vi "3D Acquisition.vi"(6 "remote cmd":T1) -> (7 "remote response":T1)   [LabVIEW 2023, in "CX Labview Wrapper.lvlib"]
uses:
  CX Labview Wrapper.lvlib
  <vilib>/userDefined/High Color/IMAQdx.ctl
  Controls/2D Camsettings.ctl
  Controls/3D Camsettings.ctl
  <extravilib>/ChannelInstances/Messenger-t'Message Queue.lvlib-Message Cluster.ctl'/))Channel.ctl
  modules/cmh-library/Message Queue/Message Cluster.ctl
  Modules/imaqdx-classes/imaqdx/C5/C5.lvclass
  D:/gitlab/thermography-acquisition/thermography-acquisition/modules/imaqdx-classes/imaqdx/Camera/GigE Camera.lvclass
  9e623b8b-350b-4dac-bc7c-d4b869b38778.vi
  5610718c-0c97-4d59-862b-e515b301dfbc.vi
  16968268-87fa-4872-9799-b0272440c818.vi
  4f413283-1e67-4ee1-b33a-2c7c3799b1f0.vi
  <extravilib>/ChannelInstances/Messenger-t'Message Queue.lvlib-Message Cluster.ctl'/Write With Abort.vi
  <extravilib>/ChannelInstances/Event Messenger-bool/Instantiate.vi
  <extravilib>/ChannelInstances/Event Messenger-bool/))Channel.vi
  <extravilib>/ChannelInstances/Messenger-t'Message Queue.lvlib-Message Cluster.ctl'/Endpoint.vi
  modules/cmh-library/Message Queue/Enqueue Multiple Messages.vi
  gitlab/thermography-acquisition/thermography-acquisition/modules/imaqdx-classes/imaqdx/Camera/Write Attributes from VArrays Cluster.vi
  Modules/cmh-library/Message Queue.lvlib
  gitlab/thermography-acquisition/thermography-acquisition/modules/imaqdx-classes/imaqdx/Camera/GigE Camera.lvclass
  modules/cmh-library/Message Queue Helper.lvlib
  <extravilib>/ChannelInstances/Event Messenger-bool.lvlib
  <vilib>/addons/_JKI.lib/Serialization/JSON/JKI JSON Serialization.lvlib
  D:/git/CX-LabVIEW-Wrapper/VI/Modules/imaqdx-classes/imaqdx/3D/3D.lvclass
  D:/git/CX-LabVIEW-Wrapper/VI/Modules/imaqdx-classes/imaqdx/C5/C5.lvclass
  <extravilib>/ChannelInstances/Messenger-t'Message Queue.lvlib-Message Cluster.ctl'.lvlib
panel:
  in  "Close Button":bool
  out "success":i32
  out "Initialized":bool
  in  "3D Cam":T2="C5"
  out "Log":string
  out "error out":errorcluster
  in  "Main Tab Control":enum32{"3D Image", "2D Image", "All Settings"}(tab)
  in  "Open 3D Image":bool caption="Open Image"
  in  "Save Pointcloud":bool
  in  "Save 3D Settings":bool caption="Save"
  in  "Apply 3D Settings":bool caption="Apply"
  in  "Channel":u16(ring) items=["DC0", "DC1", "DC2"]
  out "FrameRate":dbl caption="FrameRate [Hz]" format="%#.2g"
  out "Traversal [mm]":dbl format="%#.2g"
  in  "Acquire 3D Button":bool caption="Acquire 3D"
  in  "Save 3D Image":bool caption="Save Image"
  in  "3D Mode Camsettings":T3={"CameraMode"=0, "ProfilesPerFrame"=0, "ExposureTimeAbs"=9000, "FramePeriod"=0, "ProfileTriggerMode"=0, "OutputImageType"=0, "FIR"=FALSE, "AcquisitionMode"=0, "AcquisitionFrameCount"=0, "AOIThreshold"=0, "AOIHeight"=0, "NumSubPixel"=0, "TriggerDivider"=0, "EnableDC0"=FALSE, "EnableDC1"=FALSE, "EnableDC2"=FALSE, "Timeout"=0} {"OutputImageType" items=["Auto"=2147483647, "Grayscale (U8)"=0, "Grayscale (I16)"=1, "Grayscale (U16)"=7, "RGB (U32)"=4, "RGB (U64)"=6]; "ProfileTriggerMode" items=["Free-Run", "Camera Input1", "Camera Input2", "Encoder/Resolver Interface RS422"]; "CameraMode" items=["Image Mode (IMG)"=0, "3D FIR Peak (PEAK)"=4, "3D Center of Gravity (COG)"=3, "3D Threshold (TRSH)"=1, "3D Maximum Intensity (MAX)"=2]; "AcquisitionMode" items=["Continuous", "Single Frame", "Multiple Frame"]}
  out "Depth Image":u16[][](graph)
  in  "CalibId":string="cal0"
  in  "Save 2D Settings":bool
  out "Processed FPS":dbl
  out "Acquired FPS":dbl
  in  "2D Play Button":bool
  in  "2D Stop Button":bool
  in  "Save Image":bool
  in  "2D Mode Camsettings":T4={"CameraMode"=0, "ExposureTimeAbs"=0, "AOIThreshold"=0.0, "FramePeriod"=0, "ProfileTriggerMode"=0, "OutputImageType"=7, "AcquisitionMode"=0, "Timeout"=1000, "EnableDC0"=TRUE} {"AcquisitionMode" items=["Continuous", "Single Frame", "Multiple Frame"]; "OutputImageType" items=["Auto"=2147483647, "Grayscale (U8)"=0, "Grayscale (I16)"=1, "Grayscale (U16)"=7, "RGB (U32)"=4, "RGB (U64)"=6]; "ProfileTriggerMode" items=["Free-Run", "Camera Input1", "Camera Input2", "Encoder/Resolver Interface RS422"]; "CameraMode" items=["Image Mode (IMG)"=0, "3D FIR Peak (PEAK)"=4, "3D Center of Gravity (COG)"=3, "3D Threshold (TRSH)"=1, "3D Maximum Intensity (MAX)"=2]}
  out "Intensity Image":u16[][](graph)
  out "2D Detail Graph":u16[][](graph)
  in  "Tab Control Pams":T5(tab)
  in  "U32 Value Control":u32(slide) step=1 scale=0.0..4294967295.0 scale format="%.0e"
  in  "DBL Value Control":dbl(slide) min=0.0 max=1023.0 step=1.0 scale=0.0..1023.0
  in  "String Value Control":string
  in  "Enum Value Control":u32(ring) items=["Image Mode (IMG)", "3D FIR Peak (PEAK)", "3D Center of Gravity (COG)", "3D Threshold (TRSH)", "3D Maximum Intensity (MAX)"]
  in  "Boolean Value Control":bool
  in  "Command Value Control":bool
  in  "Attribute Tree":string(tree)
  out "Tooltip":string
  out "Units":string
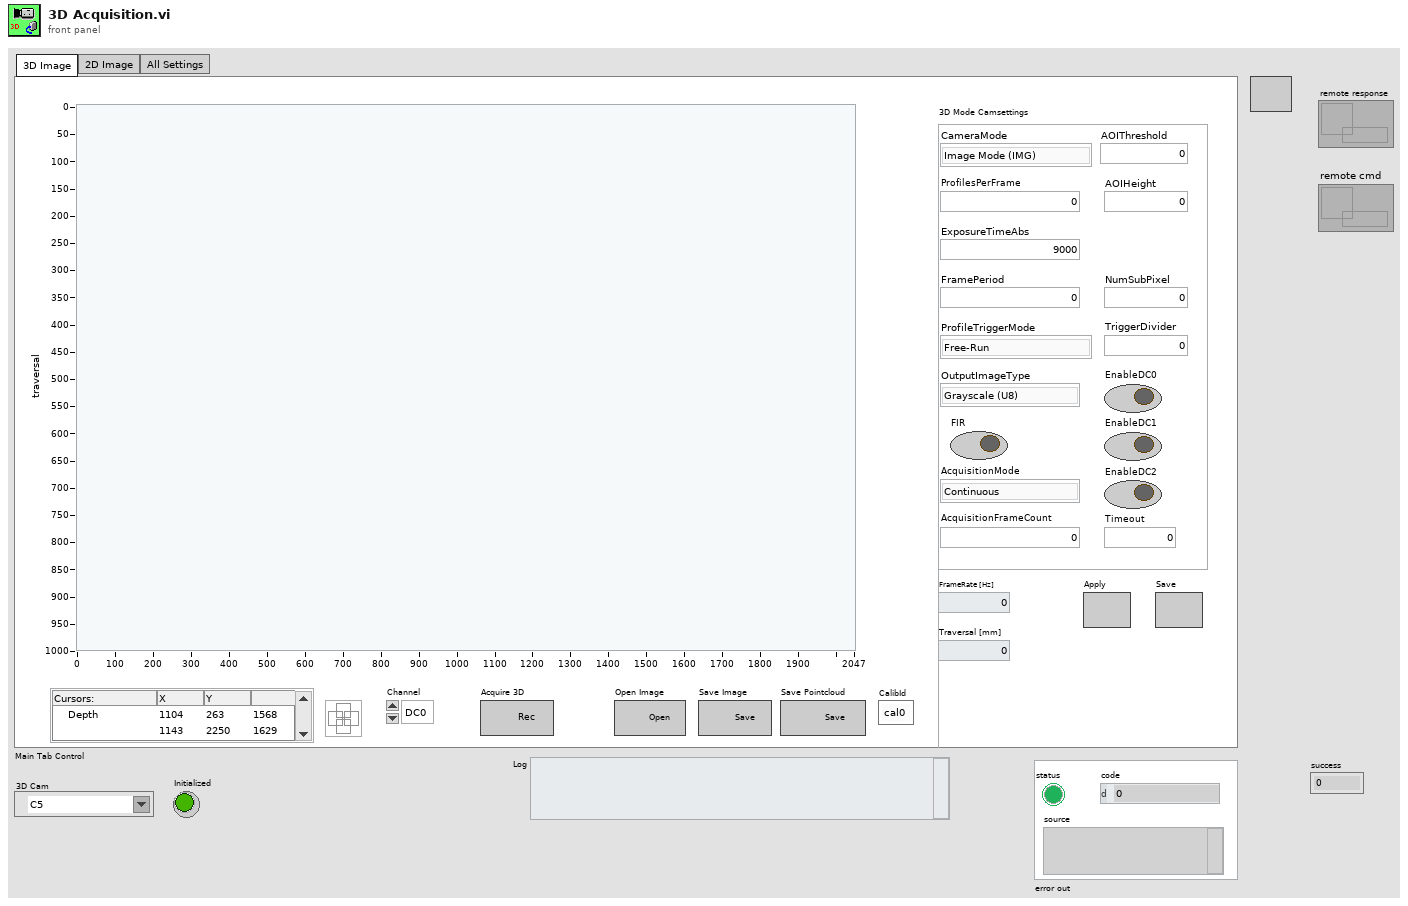
[diagram p1: front panel]
types:
  T1 = typedef "Messenger-t'Message Queue.lvlib-Message Cluster.ctl'.lvlib/))Channel.ctl" = refnum<queue>
  T2 = typedef "IMAQdx.ctl" = refnum<k21>
  T3 = typedef "CX Labview Wrapper.lvlib/3D Camsettings.ctl" = cluster{"CameraMode":u32, "ProfilesPerFrame":i64, "ExposureTimeAbs":i64, "FramePeriod":i64, "ProfileTriggerMode":u32, "OutputImageType":u32, "FIR":bool, "AcquisitionMode":u32, "AcquisitionFrameCount":i64, "AOIThreshold":i64, "AOIHeight":i64, "NumSubPixel":i64, "TriggerDivider":i64, "EnableDC0":bool, "EnableDC1":bool, "EnableDC2":bool, "Timeout":u32}
  T4 = typedef "CX Labview Wrapper.lvlib/2D Camsettings.ctl" = cluster{"CameraMode":u32, "ExposureTimeAbs":i64, "AOIThreshold":dbl, "FramePeriod":i64, "ProfileTriggerMode":u32, "OutputImageType":u32, "AcquisitionMode":u32, "Timeout":i64, "EnableDC0":bool}
  T5 = enum32{"U32", "DBL", "String", "Enum", "Bool", "Command"}
  T6 = cluster{"Element Names":string[], "Array of VData":variant[]}
  T7 = enum16{"DC0 DC2", "DC2", "DC0", "DC0 DC1 DC2", "DC1", "DC1 DC2", "DC0 DC1", ""}
  T8 = cluster{"Tab Control Pams":refnum<vi>, "U32 Value Control":refnum<vi>, "DBL Value Control":refnum<vi>, "String Value Control":refnum<vi>, "Enum Value Control":refnum<vi>, "Boolean Value Control":refnum<vi>, "Command Value Control":refnum<vi>}
  T9 = typedef "IMAQ Image.ctl" = refnum<image>
  T10 = typedef "Event Messenger-bool.lvlib/))Channel.ctl" = refnum<queue>
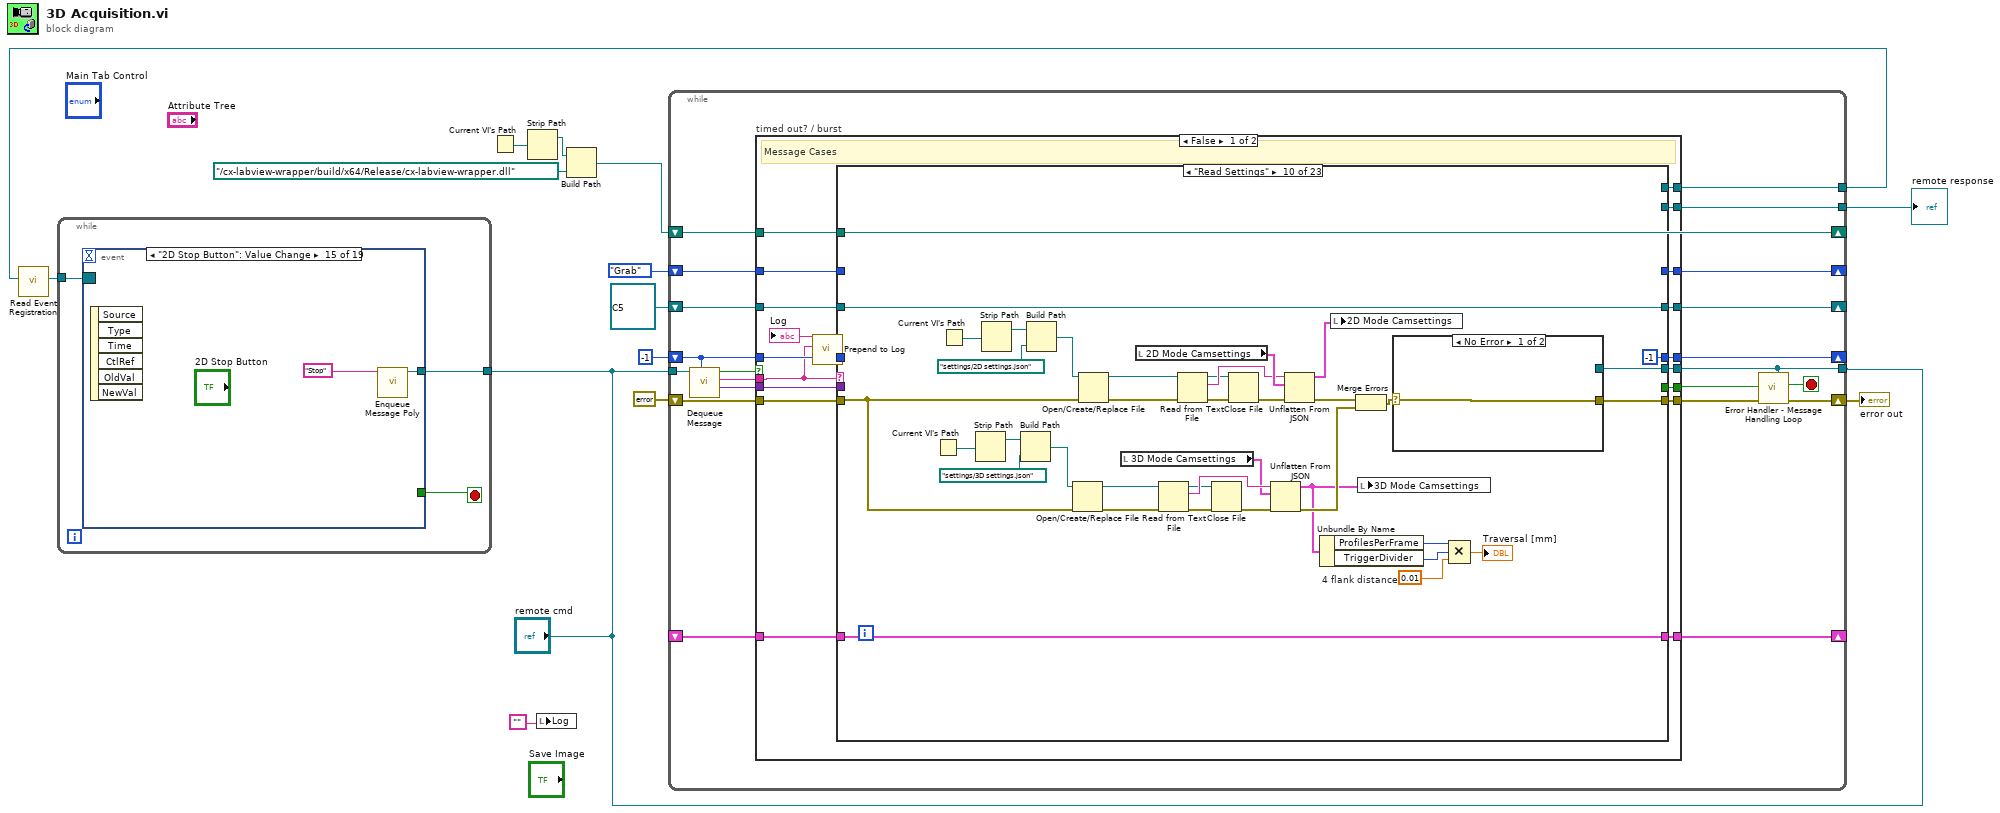
[diagram p0: block diagram]
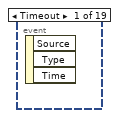
[diagram p2: hidden frame]
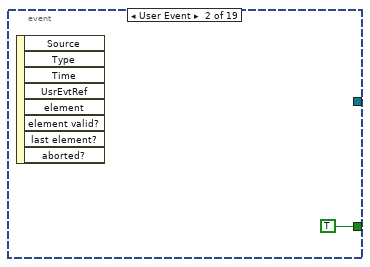
[diagram p3: hidden frame]
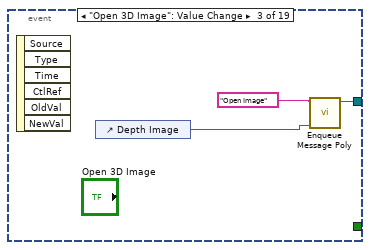
[diagram p4: hidden frame]
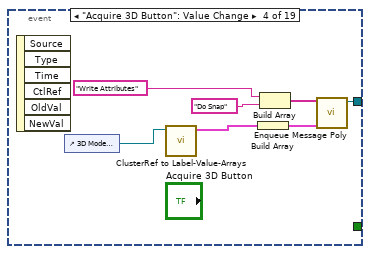
[diagram p5: hidden frame]
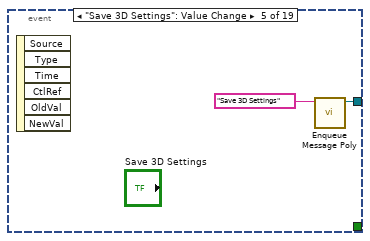
[diagram p6: hidden frame]
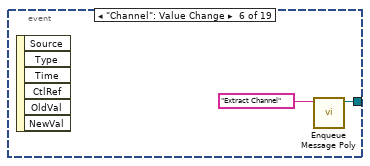
[diagram p7: hidden frame]
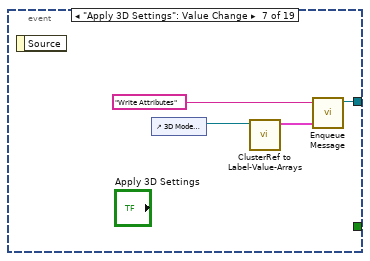
[diagram p8: hidden frame]
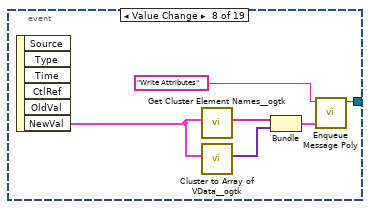
[diagram p9: hidden frame]
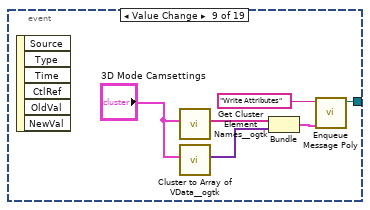
[diagram p10: hidden frame]
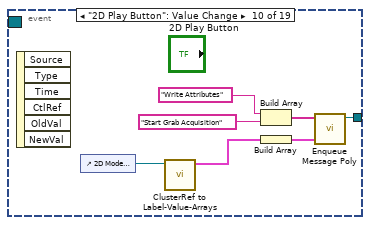
[diagram p11: hidden frame]
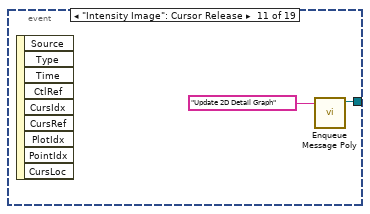
[diagram p12: hidden frame]
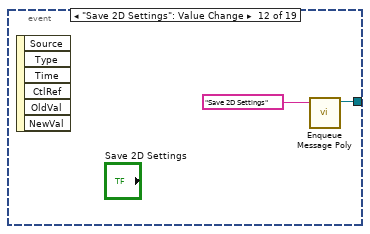
[diagram p13: hidden frame]
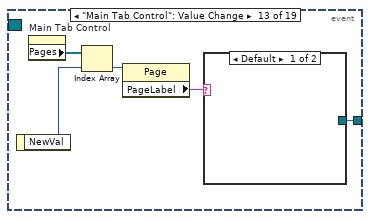
[diagram p14: hidden frame]
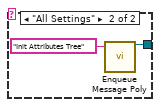
[diagram p15: hidden frame]
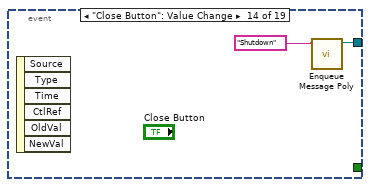
[diagram p16: hidden frame]
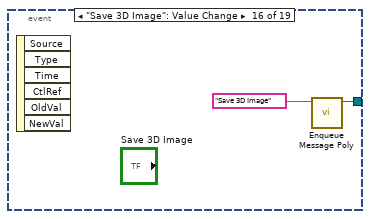
[diagram p17: hidden frame]
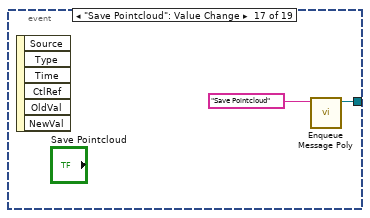
[diagram p18: hidden frame]
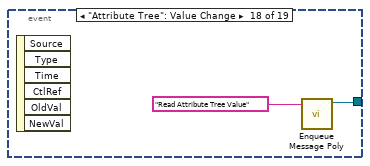
[diagram p19: hidden frame]
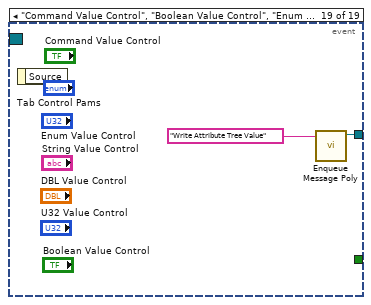
[diagram p20: hidden frame]
diagram:
  n1 = Current VI's Path() -> (path=w6:path)
  n2 = Strip Path(path=w6) -> (stripped path=w5:path)  [unwired: 1 out]
  n3 = local write "Log"("") -> ()
  n4 = Build Path(base path=w5, name or relative path=path "../cx-labview-wrapper/build/x64/Release/cx-labview-wrapper.dll") -> (appended path=w4:path)
  n5 = call <extravilib>:"Read Event Registration.vi"("channel"=w10) -> ("event registration refnum"=w9:refnum<event-registration>)  [unwired: 10 in]
  n6 = while {
    tunnel: [w17] -> w2
    tunnel: w9 -> [w16]
    stop <- w15 stop-if-true
    n7 = event shown="[14] \"2D Stop Button\": Value Change" {
      selector: w16 -> [_ _ _ _ _ _ _ _ _ _ _ _ _ _ _ _ _ _ _]
      dyn-events: _ -> [_ _ _ _ _ _ _ _ _ _ _ _ _ _ _ _ _ _ _]
      timeout: _ -> [_ _ _ _ _ _ _ _ _ _ _ _ _ _ _ _ _ _ _]
      tunnel: [_ _ w21 w27 w30 w32 w36 w42 w48 w55 w56 w58 w60 w68 w69 w72 w74 w75 w77] -> w17
      tunnel: [_ TRUE _ _ _ _ _ _ _ _ _ _ _ _ _ _ _ _ _] -> w15
      event Timeout {
        n8 = event-data() -> ()  [unwired: 1 in, 3 out]
      }
      event User Event {
        n9 = event-data() -> ()  [unwired: 1 in, 8 out]
      }
      event "Open 3D Image": Value Change {
        n10 = event-data() -> ()  [unwired: 1 in, 6 out]
        n11 = control-ref of="Depth Image"() -> (w19:refnum<vi>)
        n12 = call-poly "Enqueue Message Poly.vi"("Message Data"=w19, "Message"="Open Image") -> ("channel"=w21:T1)  [unwired: 9 in]
      }
      event "Acquire 3D Button": Value Change {
        n13 = event-data() -> ()  [unwired: 1 in, 6 out]
        n14 = control-ref of="3D Mode Camsettings"() -> (w22:refnum<vi>)
        n15 = call "ClusterRef to Label-Value-Arrays.vi"("Cluster in"=w22) -> ("Labels-Values Cluster"=w23:cluster{string[], variant[]})  [unwired: 9 in, 1 out]
        n16 = Build Array(w23) -> (w24:cluster{string[], variant[]}[])
        n17 = Build Array("Write Attributes" ("Message"), "Do Snap" ("Message")) -> (w25:string[])
        n18 = call-poly "Enqueue Message Poly.vi"("data array"=w24, "cmd array"=w25) -> ("channel"=w27:T1)  [unwired: 9 in]
      }
      event "Save 3D Settings": Value Change {
        n19 = event-data() -> ()  [unwired: 1 in, 6 out]
        n20 = call-poly "Enqueue Message Poly.vi"("Message"="Save 3D Settings") -> ("channel"=w30:T1)  [unwired: 10 in]
      }
      event "Channel": Value Change {
        n21 = event-data() -> ()  [unwired: 1 in, 6 out]
        n22 = call-poly "Enqueue Message Poly.vi"("Message"="Extract Channel") -> ("channel"=w32:T1)  [unwired: 10 in]
      }
      event "Apply 3D Settings": Value Change {
        n23 = event-data() -> ()  [unwired: 1 in, 1 out]
        n24 = control-ref of="3D Mode Camsettings"() -> (w34:refnum<vi>)
        n25 = call "ClusterRef to Label-Value-Arrays.vi"("Cluster in"=w34) -> ("Labels-Values Cluster"=w33:cluster{string[], variant[]})  [unwired: 9 in, 1 out]
        n26 = call "Enqueue Message.vi"("Message Data"=w33, "Message"="Write Attributes") -> ("channel"=w36:T1)  [unwired: 9 in]
      }
      event Value Change {
        n27 = event-data() -> ("NewVal"=w37:T4)  [unwired: 1 in, 5 out]
        n28 = call <userlib>:"Get Cluster Element Names__ogtk.vi"("Cluster"=w37) -> ("Element Names"=w40:string[])  [unwired: 9 in, 1 out]
        n29 = call <userlib>:"Cluster to Array of VData__ogtk.vi"("Cluster"=w37) -> ("Array of VData"=w39:variant[])  [unwired: 9 in, 1 out]
        n30 = Bundle("Element Names"=w40, "Array of VData"=w39) -> (w38:T6)  [unwired: 1 in]
        n31 = call-poly "Enqueue Message Poly.vi"("Message Data"=w38, "Message"="Write Attributes") -> ("channel"=w42:T1)  [unwired: 9 in]
      }
      event Value Change {
        n32 = event-data() -> ()  [unwired: 1 in, 6 out]
        n33 = call <userlib>:"Get Cluster Element Names__ogtk.vi"("Cluster"="3D Mode Camsettings") -> ("Element Names"=w45:string[])  [unwired: 9 in, 1 out]
        n34 = call <userlib>:"Cluster to Array of VData__ogtk.vi"("Cluster"="3D Mode Camsettings") -> ("Array of VData"=w44:variant[])  [unwired: 9 in, 1 out]
        n35 = Bundle("Element Names"=w45, "Array of VData"=w44) -> (w43:T6)  [unwired: 1 in]
        n36 = call-poly "Enqueue Message Poly.vi"("Message Data"=w43, "Message"="Write Attributes") -> ("channel"=w48:T1)  [unwired: 9 in]
      }
      event "2D Play Button": Value Change {
        n37 = event-data() -> ()  [unwired: 1 in, 6 out]
        n38 = control-ref of="2D Mode Camsettings"() -> (w50:refnum<vi>)
        n39 = call "ClusterRef to Label-Value-Arrays.vi"("Cluster in"=w50) -> ("Labels-Values Cluster"=w49:cluster{string[], variant[]})  [unwired: 9 in, 1 out]
        n40 = Build Array("Write Attributes" ("Message"), "Start Grab Acquisition" ("Message")) -> (w54:string[])
        n41 = Build Array(w49) -> (w51:cluster{string[], variant[]}[])
        n42 = call-poly "Enqueue Message Poly.vi"("data array"=w51, "cmd array"=w54) -> ("channel"=w55:T1)  [unwired: 9 in]
      }
      event "Intensity Image": Cursor Release {
        n43 = event-data() -> ()  [unwired: 1 in, 9 out]
        n44 = call-poly "Enqueue Message Poly.vi"("Message"="Update 2D Detail Graph") -> ("channel"=w56:T1)  [unwired: 10 in]
      }
      event "Save 2D Settings": Value Change {
        n45 = event-data() -> ()  [unwired: 1 in, 6 out]
        n46 = call-poly "Enqueue Message Poly.vi"("Message"="Save 2D Settings") -> ("channel"=w58:T1)  [unwired: 10 in]
      }
      event "Main Tab Control": Value Change {
        n47 = event-data() -> ("NewVal"=w63:enum32{"3D Image", "2D Image", "All Settings"})  [unwired: 1 in]
        n48 = property on="Main Tab Control" class="TabCtl (strict)"() -> ("Pages"=w64:refnum<vi>[])  [unwired: 2 in, 2 out]
        n49 = Index Array(array=w64, index=w63) -> (element=w62:refnum<vi>)
        n50 = property class="Page"(reference=w62) -> ("PageLabel"=w61:string)  [unwired: 1 in, 2 out]
        n51 = case shown="Default" w61 {
          tunnel: [_ w65] -> w60
          frame Default {
          }
          frame "All Settings" {
            n52 = call-poly "Enqueue Message Poly.vi"("Message"="Init Attributes Tree") -> ("channel"=w65:T1)  [unwired: 10 in]
          }
        }
      }
      event "Close Button": Value Change {
        n53 = event-data() -> ()  [unwired: 1 in, 6 out]
        n54 = call-poly "Enqueue Message Poly.vi"("Message"="Shutdown") -> ("channel"=w68:T1)  [unwired: 10 in]
      }
      event "2D Stop Button": Value Change {
        n55 = event-data() -> ()  [unwired: 1 in, 6 out]
        n56 = call-poly "Enqueue Message Poly.vi"("Message"="Stop") -> ("channel"=w69:T1)  [unwired: 10 in]
      }
      event "Save 3D Image": Value Change {
        n57 = event-data() -> ()  [unwired: 1 in, 6 out]
        n58 = call-poly "Enqueue Message Poly.vi"("Message"="Save 3D Image") -> ("channel"=w72:T1)  [unwired: 10 in]
      }
      event "Save Pointcloud": Value Change {
        n59 = event-data() -> ()  [unwired: 1 in, 6 out]
        n60 = call-poly "Enqueue Message Poly.vi"("Message"="Save Pointcloud") -> ("channel"=w74:T1)  [unwired: 10 in]
      }
      event "Attribute Tree": Value Change {
        n61 = event-data() -> ()  [unwired: 1 in, 6 out]
        n62 = call-poly "Enqueue Message Poly.vi"("Message"="Read Attribute Tree Value") -> ("channel"=w75:T1)  [unwired: 10 in]
      }
      event "Command Value Control", "Boolean Value Control", "Enum Value Control", "String Value Control", "DBL Value Control", "U32 Value Control": Value Change {
        n63 = event-data() -> ()  [unwired: 1 in, 1 out]
        n64 = call-poly "Enqueue Message Poly.vi"("Message"="Write Attribute Tree Value") -> ("channel"=w77:T1)  [unwired: 10 in]
      }
    }
  }
  "remote cmd" <- w2
  n65 = while {
    shift-right: [w92] -> _
    shift-left: refnum<class "C5.lvclass"> refnum ("Imaqdx Classes.lvlib:C5.lvclass") -> [w98]
    tunnel: w2 -> [w97]
    shift-right: [w95] -> _
    shift-left: -1 -> [w86]
    tunnel: w2 -> [w91]
    shift-right: [w93] -> _
    shift-left: enum16{"Ring", "Grab"}."Grab" -> [w94]
    tunnel: [w85] -> w10
    shift-right: [w88] -> w11
    shift-left: errorcluster {"status"=FALSE, "code"=0, "source"=""} ("error constant") -> [w99]
    shift-right: [w83] -> _
    shift-left: _ -> [w82]
    shift-right: [w80] -> _
    shift-left: w4 -> [w80]
    tunnel: [w79] -> w1
    stop <- w89 stop-if-true
    n66 = call "Dequeue Message.vi"("timeout in ms (-1)"=w86, "channel"=w97) -> ("message data"=w96:variant, "message"=w84:string, "timed out?"=w87:bool)  [unwired: 7 in]
    n67 = case "timed out? / burst" shown="False" w87 {
      tunnel: w99 -> [w117 w550]
      tunnel: w98 -> [w116 w546]
      tunnel: [w109 w549] -> w81
      tunnel: [w115 _] -> w90
      tunnel: w96 -> [w114 _]
      tunnel: w84 -> [w104 _]
      tunnel: [w113 w544] -> w95
      tunnel: w94 -> [w108 w548]
      tunnel: [w112 w547] -> w93
      tunnel: [w111 w545] -> w92
      tunnel: [w110 w543] -> w91
      tunnel: w86 -> [w107 _]
      tunnel: [w106 _] -> w85
      tunnel: [w103 w542] -> w83
      tunnel: w82 -> [w102 w542]
      tunnel: w80 -> [w101 _]
      tunnel: [w100 _] -> w79
      frame False {
        # "Message Cases"
        n68 = call "Prepend to Log.vi"("new entry"=w104) -> ("Log out"=→"Log":string)  [unwired: 10 in]
        n69 = case shown="\"Read Settings\"" w104 {
          selector: w104 -> [_ _ _ _ _ _ _ _ _ _ _ _ _ _ _ _ _ _ _ _ _ _ w534]
          tunnel: w114 -> [_ _ _ _ _ _ w234 _ _ _ _ _ w342 _ _ _ _ _ _ _ _ w530 _]
          tunnel: w117 -> [w119 w127 w146 w161 w179 w203 w238 w242 w256 w267 w313 w333 w358 w391 w401 w418 w462 w467 w477 w482 w498 w531 w537]
          tunnel: w116 -> [w121 w125 w149 w160 w175 w198 w240 w241 w257 w295 w318 w336 w361 w395 w402 w428 w460 w464 w479 w490 w495 w512 w540]
          tunnel: [_ _ _ _ _ _ _ _ _ _ _ _ _ _ _ _ TRUE _ _ _ _ _ _] -> w115
          tunnel: [-1 ("repeat") -1 ("repeat") -1 ("repeat") -1 ("repeat") -1 ("repeat") -1 ("repeat") -1 ("repeat") w250 -1 ("repeat") -1 ("repeat") -1 ("repeat") -1 ("repeat") -1 ("repeat") -1 ("repeat") 0 ("repeat") -1 ("repeat") -1 ("repeat") 0 ("repeat") -1 ("repeat") w484 w492 -1 ("repeat") -1 ("repeat")] -> w113
          tunnel: [_ _ _ _ _ _ _ _ _ _ _ _ _ _ enum16{"Ring", "Grab"}."Grab" _ w458 enum16{"Ring", "Grab"}."Grab" _ w485 w494 _ w539] -> w112
          tunnel: [w121 w125 w149 w160 w174 w197 w240 w248 w257 w295 w318 w336 w361 w395 w398 w428 w459 w469 w475 w490 w495 w512 w540] -> w111
          tunnel: [_ w128 w144 _ _ w200 _ _ _ w278 _ _ _ _ _ _ _ _ _ _ _ _ _] -> w110
          tunnel: [w119 w129 w146 w159 w181 w201 w236 w249 w253 w289 w309 w324 w351 w387 w404 w414 w454 w471 w476 w487 w496 w503 w536] -> w109
          tunnel: w108 -> [_ _ _ _ _ _ _ _ _ _ _ _ _ _ _ _ w458 _ _ w485 w494 _ w539]
          tunnel: w107 -> [_ _ _ _ _ _ _ _ _ _ _ _ _ _ _ _ _ _ _ w484 w492 _ _]
          tunnel: [_ _ _ _ _ _ _ _ _ _ _ _ _ _ _ _ w452 _ _ _ _ _ _] -> w106
          tunnel: [w118 w131 w147 w169 w182 w189 w237 w247 w251 w293 w316 w334 w359 w393 w396 w435 w451 w472 w474 w491 w493 w529 w538] -> w103
          tunnel: w102 -> [w118 w131 w147 w169 w182 _ w237 w247 w251 w293 w316 w334 w359 w393 w396 w435 w451 w472 w474 w491 w493 w529 w538]
          tunnel: w101 -> [_ _ _ _ _ _ _ _ _ _ _ w330 w356 _ _ w413 _ _ _ _ _ _ _]
          tunnel: [_ _ _ _ _ w184 _ _ _ _ _ _ _ _ _ _ _ _ _ _ _ _ _] -> w100
          frame "-COPY THIS FRAME-" {
          }
          frame "Do Snap" {
            n70 = local read "3D Mode Camsettings"() -> (w123:T3)
            n71 = call-dynamic "Reset AOI.vi"("error in (no error)"=w127, "C5 in"=w125) -> ("error out"=w126:errorcluster, "C5 out"=w124:refnum<class "C5.lvclass">)  [unwired: 8 in]
            n72 = Unbundle By Name(w123) -> ("Timeout"=w122:u32)
            n73 = call-dynamic "Do Snap.vi"("error in (no error)"=w126, "Timeout (ms)"=w122, "GigE Camera in"=w124) -> ("error out"=w130:errorcluster)  [unwired: 6 in, 2 out]
            n74 = case shown="No Error" w130 {
              selector: w130 -> [w135 w136]
              tunnel: [w135 w136] -> w129
              tunnel: [w133 _] -> w128
              frame No Error {
                n75 = call-poly "Enqueue Message Poly.vi"("Message"="Extract Channel") -> ("channel"=w133:T1)  [unwired: 10 in]
              }
              frame Error {
              }
            }
          }
          frame "Error" {
            n76 = Unbundle By Name(w146) -> ("code"=w142:i32, "source"=w139:string)
            n77 = Format Into String(format string="%d", w142) -> (resulting string=w141:string)  [unwired: 2 in, 1 out]
            n78 = call <vilib>:"Space Constant.vi"() -> ("String"=w140:string)
            n79 = Concatenate Strings(w141, w140, w139) -> (w138:string)
            n80 = call "Prepend to Log.vi"("new entry"=w138) -> ("Log out"=w145:string)  [unwired: 10 in]
            n81 = local write "Log"(w145) -> ()
            n82 = call-poly "Enqueue Message Poly.vi"("Message"="Shutdown") -> ("channel"=w144:T1)  [unwired: 10 in]
          }
          frame "Extract Channel" {
            # "connect this to settings"
            n83 = call "Seperate Channels.vi"("Output"=T7."DC0 DC2", "error in (no error)"=w161, "C5 in"=w160) -> ("error out"=w163:errorcluster, "DC2"=w167:u16[][], "DC1"=w165:u16[][], "DC0"=w164:u16[][])  [unwired: 5 in]
            n84 = case shown="0, Default" "Channel" {
              tunnel: w167 -> [_ _ w173]
              tunnel: [w171 w172 w173] -> w157
              tunnel: w165 -> [_ w172 _]
              tunnel: w164 -> [w171 _ _]
              frame 0, Default {
              }
              frame 1 {
              }
              frame 2 {
              }
            }
            n85 = Transpose 2D Array(2D array=w157) -> (transposed array=→"Depth Image":u16[][])
            n86 = Array Size(array=w157) -> (size(s)=w156:i32[])
            n87 = Index Array(array=w156) -> (element #1=w155:i32, element #2=w153:i32)  [unwired: 2 in]
            n88 = control-ref of="Depth Image"() -> (w158:refnum<vi>)
            n89 = Decrement(x=w155) -> (x-1=w154:i32)
            n90 = Decrement(x=w153) -> (x-1=w152:i32)
            n91 = property class="IntGraph (strict)"(reference=w158, error in=w163, "YScale.Maximum"=w154, "XScale.Maximum"=w152, "YScale.Minimum"=0.0 ("Y Scale.Range:Minimum"), "XScale.Minimum"=0.0 ("X Scale.Range:Minimum")) -> (error out=w159:errorcluster)  [unwired: 1 out]
          }
          frame "Init Attributes Tree" {
            n92 = call "Stop Acquisition.vi"("error in (no error)"=w179, "GigE Camera in"=w175) -> ("error out"=w178:errorcluster, "GigE Camera out"=w177:refnum<class "C5.lvclass">)  [unwired: 8 in]
            n93 = call-dynamic "Unconfigure Acquisition.vi"("error in (no error)"=w178, "GigE Camera in"=w177) -> ("error out"=w176:errorcluster, "GigE Camera out"=w174:refnum<class "C5.lvclass">)  [unwired: 8 in]
            n94 = control-ref of="Attribute Tree"() -> (w180:refnum<vi>)
            n95 = call-dynamic "Init Attributes Tree.vi"("error in (no error)"=w176, "Tree Control In"=w180, "GigE Camera in"=w174) -> ("error out"=w181:errorcluster)  [unwired: 6 in, 2 out]
          }
          frame "Init" {
            n96 = property on="Intensity Image" class="IntGraph (strict)"("ZScale.MarkerVals[]"=cluster{u16, u32}[] [{0, 0}, {1023, 16448250}] ("Z Scale.Marker Values[]")) -> ()  [unwired: 2 in, 2 out]
            n97 = property on="Initialized" class="Bool (strict)"(error in=w203, "Value"=FALSE ("Initialized")) -> (error out=w188:errorcluster)  [unwired: 1 in, 1 out]
            n98 = control-ref of="Boolean Value Control"() -> (w191:refnum<vi>)
            n99 = control-ref of="String Value Control"() -> (w193:refnum<vi>)
            n100 = control-ref of="U32 Value Control"() -> (w195:refnum<vi>)
            n101 = control-ref of="DBL Value Control"() -> (w194:refnum<vi>)
            n102 = control-ref of="Enum Value Control"() -> (w192:refnum<vi>)
            n103 = control-ref of="Command Value Control"() -> (w190:refnum<vi>)
            n104 = control-ref of="Tab Control Pams"() -> (w196:refnum<vi>)
            n105 = call-dynamic "Init Cam.vi"("error in (no error)"=w188, "Camera Name"="3D Cam", "Camera in"=w198) -> ("error out"=w199:errorcluster, "Camera out"=w197:refnum<class "C5.lvclass">)  [unwired: 7 in]
            n106 = Unbundle By Name(w199) -> ("code"=w202:i32)
            n107 = Bundle("Tab Control Pams"=w196, "U32 Value Control"=w195, "DBL Value Control"=w194, "String Value Control"=w193, "Enum Value Control"=w192, "Boolean Value Control"=w191, "Command Value Control"=w190) -> (w189:T8)  [unwired: 1 out]
            n108 = case shown="0" w202 {
              selector: w202 -> [w210 _ _ _]
              tunnel: w199 -> [w212 w219 w226 w229]
              tunnel: [w211 w219 w225 w228] -> w201
              tunnel: [w207 w217 w224 w227] -> w200
              tunnel: [_ _ w220 _] -> w184
              frame Default {
                n109 = Format Into String(format string="%d", initial string="code: ", error in=w212, w210) -> (resulting string=w205:string, error out=w211:errorcluster)
                n110 = call-poly "Enqueue Message Poly.vi"("Message Data"=w205, "Message"="Log") -> ("channel"=w207:T1)  [unwired: 9 in]
              }
              frame 0 {
                n111 = Build Array("Populate Settings Controls" ("Message"), "Read Settings" ("Message"), "Init Attributes Tree" ("Message")) -> (w215:string[])
                n112 = call-poly "Enqueue Message Poly.vi"("cmd array"=w215) -> ("channel"=w217:T1)  [unwired: 10 in]
                "Initialized" <- TRUE ("Initialized")
              }
              frame -1074360311 {
                w222 = "Log" ("Message")
                n113 = call <vilib>:"Clear Errors.vi"("error in (no error)"=w226) -> ("error out"=w225:errorcluster)  [unwired: 5 in, 1 out]
                n114 = call-poly "Enqueue Message Poly.vi"("Message Data"="Warning: Cam not found" ("Message"), "Message"=w222) -> ("channel"=w224:T1)  [unwired: 9 in]
                n115 = call-poly "Enqueue Message Poly.vi"("Message Data"="3D Module - Warning: Cam not found" ("Message"), "Message"=w222) -> ("channel"=w220:T1)  [unwired: 9 in]
              }
              frame -1074360310 {
                n116 = call <vilib>:"Clear Errors.vi"("error in (no error)"=w229) -> ("error out"=w228:errorcluster)  [unwired: 5 in, 1 out]
                n117 = call-poly "Enqueue Message Poly.vi"("Message Data"="Warning: Cam already in use" ("Message"), "Message"="Log") -> ("channel"=w227:T1)  [unwired: 9 in]
              }
            }
          }
          frame "Log" {
            n118 = call "Variant to Data.vim"("variant"=w234, "type"="", "Error In"=w238) -> ("data"=w233:string, "Error Out"=w236:errorcluster)  [unwired: 11 in]
            n119 = call "Prepend to Log.vi"("new entry"=w233) -> ("Log out"=w232:string)  [unwired: 10 in]
            n120 = local write "Log"(w232) -> ()
          }
          frame "Populate Settings Controls" {
            w250 = -1  # default
            n121 = control-ref of="3D Mode Camsettings"() -> (w244:refnum<vi>)
            n122 = call-dynamic "Populate Settings.vi"("error in (no error)"=w242, "Settings Cluster"=w244, "GigE Camera in"=w241) -> ("error out"=w245:errorcluster, "GigE Camera out"=w243:refnum<class "C5.lvclass">)  [unwired: 7 in]
            n123 = control-ref of="2D Mode Camsettings"() -> (w246:refnum<vi>)
            n124 = call-dynamic "Populate Settings.vi"("error in (no error)"=w245, "Settings Cluster"=w246, "GigE Camera in"=w243) -> ("error out"=w249:errorcluster, "GigE Camera out"=w248:refnum<class "C5.lvclass">)  [unwired: 7 in]
          }
          frame "Read Attribute Tree Value" {
            n125 = control-ref of="Attribute Tree"() -> (w252:refnum<vi>)
            n126 = call-dynamic "Read Attribute Tree Value.vi"("error in (no error)"=w256, "Controls Cluster"=w251, "Attribute Tree"=w252, "GigE Camera in"=w257) -> ("error out"=w253:errorcluster, "Tooltip"=→"Tooltip":string, "Units"=→"Units":string)  [unwired: 4 in, 1 out]
          }
          frame "Read Settings" {
            w260 = 0.01  # 4 flank distance
            n127 = Current VI's Path() -> (path=w277:path)
            n128 = Current VI's Path() -> (path=w292:path)
            n129 = Strip Path(path=w277) -> (stripped path=w276:path)  [unwired: 1 out]
            n130 = Strip Path(path=w292) -> (stripped path=w291:path)  [unwired: 1 out]
            n131 = Build Path(base path=w276, name or relative path=path "settings/3D settings.json" ("Relative path (.)")) -> (appended path=w274:path)
            n132 = Build Path(base path=w291, name or relative path=path "settings/2D settings.json" ("Relative path (.)")) -> (appended path=w287:path)
            n133 = Open/Create/Replace File(file path (use dialog)=w274, error in=w267) -> (refnum out=w273:refnum<file>, error out=w268:errorcluster)  [unwired: 4 in, 1 out]
            n134 = Open/Create/Replace File(file path (use dialog)=w287, error in=w267) -> (refnum out=w286:refnum<file>, error out=w288:errorcluster)  [unwired: 4 in, 1 out]
            n135 = local read "3D Mode Camsettings"() -> (w259:T3)
            n136 = local read "2D Mode Camsettings"() -> (w285:T4)
            n137 = Read from Text File(file (use dialog)=w273, error in=w268) -> (refnum out=w271:refnum<file>, text=w272:string, error out=w269:errorcluster)  [unwired: 2 in, 1 out]
            n138 = Read from Text File(file (use dialog)=w286, error in=w288) -> (refnum out=w280:refnum<file>, text=w283:string, error out=w282:errorcluster)  [unwired: 2 in, 1 out]
            n139 = Close File(refnum=w271, error in=w269) -> (error out=w270:errorcluster)  [unwired: 1 out]
            n140 = Close File(refnum=w280, error in=w282) -> (error out=w281:errorcluster)  [unwired: 1 out]
            n141 = Unflatten From JSON(JSON string=w272, type and defaults=w259, error in (no error)=w270) -> (value=w264:T3, error out=w265:errorcluster)  [unwired: 4 in]
            n142 = Unflatten From JSON(JSON string=w283, type and defaults=w285, error in (no error)=w281) -> (value=w284:T4, error out=w279:errorcluster)  [unwired: 4 in]
            n143 = Unbundle By Name(w264) -> ("ProfilesPerFrame"=w262:i64, "TriggerDivider"=w261:i64)
            n144 = local write "2D Mode Camsettings"(w284) -> ()
            n145 = Merge Errors(w279, w265) -> (w266:errorcluster)
            n146 = local write "3D Mode Camsettings"(w264) -> ()
            n147 = case shown="No Error" w266 {
              selector: w266 -> [w296 w302]
              tunnel: [w296 w301] -> w289
              tunnel: [_ w300] -> w278
              frame No Error {
              }
              frame Error {
                n148 = call <vilib>:"Clear Errors.vi"("error in (no error)"=w302, "specific error code to clear (0: all)"=-375006) -> ("error out"=w301:errorcluster)  [unwired: 4 in, 1 out]
                n149 = call-poly "Enqueue Message Poly.vi"("Message Data"="Warning: Unflatten from JSON" ("Message"), "Message"="Log") -> ("channel"=w300:T1)  [unwired: 9 in]
              }
            }
            n150 = Compound Arithmetic op=MULTIPLY(w262, w261, w260) -> (→"Traversal [mm]":dbl)
          }
          frame "Save 2D Settings" {
            n151 = Current VI's Path() -> (path=w307:path)
            n152 = Strip Path(path=w307) -> (stripped path=w306:path)  [unwired: 1 out]
            n153 = call <vilib>:"Flatten To JSON String.vi"("error in (no error)"=w313, "Variant"="2D Mode Camsettings") -> ("error out"=w314:errorcluster, "JSON String"=w311:string)  [unwired: 8 in]
            n154 = Build Path(base path=w306, name or relative path=path "settings/2D settings.json" ("Relative path (.)")) -> (appended path=w304:path)
            n155 = Open/Create/Replace File(file path (use dialog)=w304, error in=w314) -> (refnum out=w303:refnum<file>, error out=w312:errorcluster)  [unwired: 4 in, 1 out]
            n156 = Write to Text File(file (use dialog)=w303, text=w311, error in=w312) -> (refnum out=w308:refnum<file>, error out=w310:errorcluster)  [unwired: 1 in, 1 out]
            n157 = Close File(refnum=w308, error in=w310) -> (error out=w309:errorcluster)  [unwired: 1 out]
          }
          frame "Save 3D Image" {
            # "int32_t writeTif_U16\n(char* file, Arr2D_U16Hdl arr)"
            n158 = Get Date/Time In Seconds() -> (seconds since 1Jan1904=w322:timestamp)
            n159 = Format Date/Time String(time format string (%c)="%d%M%y%h%m", seconds (now)=w322) -> (date/time string=w320:string)  [unwired: 1 in]
            n160 = Concatenate Strings(w320, ".tif" ("string")) -> (w319:string)
            n161 = local read "Depth Image"() -> (w332:u16[][])
            n162 = call "File Dialog"("default name"=w319, "error in"=w333) -> ("selected path"=w329:path, "error out"=w331:errorcluster)  [unwired: 10 in, 2 out]
            n163 = Path To String(path=w329) -> (string=w328:string)
            n164 = Transpose 2D Array(2D array=w332) -> (transposed array=w327:u16[][])
            n165 = dll-call lib="?" fn="writeTif_U16"(path in=w330, error in=w331, "tifFile"=w328, "rangeImage"=w327) -> (error out=w325:errorcluster, "success"=w326:i32)  [unwired: 3 in, 1 out]
            n166 = case shown="1" w326 {
              tunnel: w325 -> [w337 w341]
              tunnel: [w337 w340] -> w324
              frame 0, Default {
              }
              frame 1 {
                n167 = call <vilib>:"Error Cluster From Error Code.vi"("error in (no error)"=w341, "error message (\"\")"="writeTif_U16" ("error message (\"\")"), "error code (0)"=5002) -> ("error out"=w340:errorcluster)  [unwired: 6 in]
              }
            }
          }
          frame "Open Image" {
            # "int32_t readTif_U16\n(char* file, Arr2D_U16Hdl arr)"
            n168 = Variant To Data(error in=w358, type=refnum<vi> refnum ("Depth Image"), Variant=w342) -> (data=w343:refnum<vi>, error out=w345:errorcluster)
            n169 = call "File Dialog2"("prompt"="Select U16 bit Range Image to Open", "error in"=w345, "pattern (all files)"="*.tif;*.tiff") -> ("selected path"=w355:path, "error out"=w357:errorcluster)  [unwired: 9 in, 2 out]
            n170 = Path To String(path=w355) -> (string=w354:string)
            n171 = dll-call lib="?" fn="readTif_U16"(path in=w356, error in=w357, "tifFile"=w354, "rangeImage"=u16[][] []) -> (error out=w352:errorcluster, "success"=w353:i32, "rangeImage"=w346:u16[][])  [unwired: 2 in, 1 out]
            n172 = Transpose 2D Array(2D array=w346) -> (transposed array=w350:u16[][])
            n173 = case shown="0, Default" w353 {
              tunnel: w352 -> [w374 w379]
              tunnel: [w375 w378] -> w351
              tunnel: w346 -> [w363 _]
              tunnel: w343 -> [w367 _]
              frame 0, Default {
                n174 = Array Size(array=w363) -> (size(s)=w373:i32[])
                n175 = Array Max & Min(array=w363) -> (max value=w362:u16)  [unwired: 3 out]
                n176 = Index Array(array=w373, index #1=0 ("index"), index #2=1 ("index")) -> (element #1=w372:i32, element #2=w371:i32)
                n177 = Decrement(x=w371) -> (x-1=w368:i32)
                n178 = Decrement(x=w372) -> (x-1=w369:i32)
                n179 = property on="Property Node" class="IntGraph (strict)"(reference=w367, error in=w374, "YScale.Maximum"=w369, "XScale.Maximum"=w368, "XScale.Minimum"=0.0 ("X Scale.Range:Minimum"), "YScale.Minimum"=0.0 ("Y Scale.Range:Minimum"), "ZScale.Maximum"=w362) -> (error out=w375:errorcluster)  [unwired: 1 out]
              }
              frame 1 {
                n180 = call <vilib>:"Error Cluster From Error Code.vi"("error in (no error)"=w379, "error message (\"\")"="readTif_U16" ("error message (\"\")"), "error code (0)"=5002) -> ("error out"=w378:errorcluster)  [unwired: 6 in]
              }
            }
            n181 = local write "Depth Image"(w350) -> ()
          }
          frame "Save 3D Settings" {
            n182 = local read "3D Mode Camsettings"() -> (w380:T3)
            n183 = Current VI's Path() -> (path=w385:path)
            n184 = Strip Path(path=w385) -> (stripped path=w384:path)  [unwired: 1 out]
            n185 = call <vilib>:"Flatten To JSON String.vi"("error in (no error)"=w391, "Variant"=w380) -> ("error out"=w392:errorcluster, "JSON String"=w389:string)  [unwired: 8 in]
            n186 = Build Path(base path=w384, name or relative path=path "settings/3D settings.json" ("Relative path (.)")) -> (appended path=w382:path)
            n187 = Open/Create/Replace File(file path (use dialog)=w382, error in=w392) -> (refnum out=w381:refnum<file>, error out=w390:errorcluster)  [unwired: 4 in, 1 out]
            n188 = Write to Text File(file (use dialog)=w381, text=w389, error in=w390) -> (refnum out=w386:refnum<file>, error out=w388:errorcluster)  [unwired: 1 in, 1 out]
            n189 = Close File(refnum=w386, error in=w388) -> (error out=w387:errorcluster)  [unwired: 1 out]
          }
          frame "Save Free Image" {
            n190 = Get Date/Time In Seconds() -> (seconds since 1Jan1904=w410:timestamp)
            n191 = call-dynamic "Get IMAQ Image Buffer.vi"("error in (no error)"=w401, "GigE Camera in"=w402) -> ("error out"=w400:errorcluster, "Image"=w399:T9, "GigE Camera out"=w398:refnum<class "C5.lvclass">)  [unwired: 7 in]
            n192 = Format Date/Time String(time format string (%c)="%M%d%H%m%S", seconds (now)=w410) -> (date/time string=w408:string)  [unwired: 1 in]
            n193 = Concatenate Strings(w408, "height.png" ("string")) -> (w407:string)
            n194 = call "File Dialog"("default name"=w407, "error in"=w400) -> ("selected path"=w403:path, "error out"=w405:errorcluster)  [unwired: 10 in, 2 out]
            n195 = call-poly "IMAQ Write File 2"("error in (no error)"=w405, "Image Quality"=u32 1000, "File Path"=w403, "Image"=w399) -> ("error out"=w404:errorcluster)  [unwired: 6 in, 1 out]
          }
          frame "Save Pointcloud" {
            n196 = Get Date/Time In Seconds() -> (seconds since 1Jan1904=w431:timestamp)
            n197 = Format Date/Time String(time format string (%c)="%d%M%y%h%m", seconds (now)=w431) -> (date/time string=w429:string)  [unwired: 1 in]
            n198 = Concatenate Strings(w429, ".ply" ("string")) -> (w433:string)
            n199 = call "File Dialog CalibFile"("prompt"="Select Calibration File", "pattern (all files)"="*.xml") -> ("selected path"=w419:path, "cancelled"=w421:bool, "error out"=w416:errorcluster)  [unwired: 10 in, 1 out]
            n200 = call "File Dialog PCD"("prompt"="Save Pointcloud File", "default name"=w433, "pattern (all files)"="*.ply") -> ("selected path"=w420:path, "cancelled"=w423:bool, "error out"=w415:errorcluster)  [unwired: 9 in, 1 out]
            n201 = Merge Errors(w418, w416, w415) -> (w417:errorcluster)
            n202 = Compound Arithmetic op=OR(w421, w423) -> (w422:bool)
            n203 = case "Dialog cancelled?" shown="False" w422 {
              tunnel: [w447 2 ("success")] -> w434
              tunnel: w420 -> [w446 _]
              tunnel: w419 -> [w443 _]
              tunnel: w417 -> [w441 w449]
              tunnel: [w440 w449] -> w414
              tunnel: w413 -> [w437 _]
              frame False {
                # "int32_t createPointcloud\n(char *calibId, char *calibFile, char *pcdFile, Arr2D_U16Hdl arr)"
                n204 = local read "Depth Image"() -> (w438:u16[][])
                n205 = Path To String(path=w443) -> (string=w442:string)
                n206 = Path To String(path=w446) -> (string=w445:string)
                n207 = Transpose 2D Array(2D array=w438) -> (transposed array=w439:u16[][])
                n208 = dll-call lib="?" fn="createPointcloud"(path in=w437, error in=w441, "calibId"="CalibId", "calibFile"=w442, "pcdFile"=w445, "rangeImage"=w439) -> (error out=w440:errorcluster, "success"=w447:i32)  [unwired: 5 in, 1 out]
              }
              frame True {
              }
            }
            "success" <- w434
          }
          frame "Shutdown" {
            n209 = call "Stop Acquisition.vi"("error in (no error)"=w462, "GigE Camera in"=w460) -> ("error out"=w461:errorcluster, "GigE Camera out"=w456:refnum<class "C5.lvclass">)  [unwired: 8 in]
            n210 = call-dynamic "Release Buffers.vi"("error in (no error)"=w461, "GigE Camera in"=w456) -> ("error out"=w457:errorcluster, "GigE Camera out"=w455:refnum<class "C5.lvclass">)  [unwired: 8 in]
            n211 = call-dynamic "Close Cam.vi"("error in (no error)"=w457, "Camera in"=w455) -> ("error out"=w454:errorcluster, "Camera out"=w459:refnum<class "C5.lvclass">)  [unwired: 8 in]
            n212 = call <extravilib>:"Write.vi"("element"=TRUE) -> ("channel"=w452:T10)  [unwired: 9 in, 1 out]
          }
          frame "Start Grab Acquisition" {
            n213 = call-dynamic "Reset AOI.vi"("error in (no error)"=w467, "C5 in"=w464) -> ("error out"=w466:errorcluster, "C5 out"=w465:refnum<class "C5.lvclass">)  [unwired: 8 in]
            n214 = call-dynamic "Configure Grab Acquisition.vi"("error in (no error)"=w466, "Number of Buffers"=u32 50, "GigE Camera in"=w465) -> ("error out"=w471:errorcluster, "GigE Camera out"=w469:refnum<class "C5.lvclass">)  [unwired: 7 in]
          }
          frame "Stop" {
            n215 = call "Stop Acquisition.vi"("error in (no error)"=w477, "GigE Camera in"=w479) -> ("error out"=w476:errorcluster, "GigE Camera out"=w475:refnum<class "C5.lvclass">)  [unwired: 8 in]
          }
          frame "Update 2D Detail Graph" {
            n216 = local read "2D Mode Camsettings"() -> (w483:T4)
            n217 = control-ref of="2D Detail Graph"() -> (w481:refnum<vi>)
            n218 = control-ref of="Intensity Image"() -> (w486:refnum<vi>)
            n219 = local read "Intensity Image"() -> (w489:u16[][])
            n220 = Unbundle By Name(w483) -> ("AOIThreshold"=w480:dbl)
            n221 = call "Graph under Cursor (SubVI).vi"("AOIThreshold"=w480, "error in (no error)"=w482, "Detail Graph"=w481, "Intensity Graph"=w486, "Intensity Image"=w489) -> ("error out"=w487:errorcluster, "Intensity under Cursor"=→"2D Detail Graph":u16[][])  [unwired: 5 in]
          }
          frame "Write Attribute Tree Value" {
            n222 = control-ref of="Attribute Tree"() -> (w497:refnum<vi>)
            n223 = call-dynamic "Write Attribute Tree Value.vi"("error in (no error)"=w498, "Value Controls Cluster"=w493, "Tree Control In"=w497, "GigE Camera in"=w495) -> ("error out"=w496:errorcluster)  [unwired: 6 in, 1 out]
          }
          frame "Write Attributes" {
            w524 = 0.01  # 4 flank distance
            # "if connected"
            n224 = call "Variant to Data.vim"("variant"=w530, "type"=T6 {"Element Names"=[], "Array of VData"=[]} ("output cluster"), "Error In"=w531) -> ("data"=w520:T6, "Error Out"=w527:errorcluster)  [unwired: 11 in]
            n225 = local read "3D Mode Camsettings"() -> (w522:T3)
            n226 = call "Stop Acquisition.vi"("error in (no error)"=w527, "GigE Camera in"=w512) -> ("error out"=w502:errorcluster, "GigE Camera out"=w501:refnum<class "C5.lvclass">)  [unwired: 8 in]
            n227 = call-dynamic "Unconfigure Acquisition.vi"("error in (no error)"=w502, "GigE Camera in"=w501) -> ("error out"=w499:errorcluster, "GigE Camera out"=w500:refnum<class "C5.lvclass">)  [unwired: 8 in]
            n228 = Unbundle By Name(w522) -> ("ProfilesPerFrame"=w526:i64, "TriggerDivider"=w525:i64)
            n229 = call-poly "Write Attributes Poly.vi"("error in (no error)"=w499, "Attributes"=w520, "GigE Camera in"=w500) -> ("error out"=w511:errorcluster, "GigE Camera out"=w518:refnum<class "C5.lvclass">)  [unwired: 7 in]
            n230 = call "Read Attribute.vi"("error in (no error)"=w511, "Attribute"="FrameRate", "GigE Camera in"=w518) -> ("error out"=w517:errorcluster, "Attribute Variant"=w516:variant)  [unwired: 5 in, 2 out]
            n231 = call "Read Attribute.vi"("error in (no error)"=w511, "Attribute"="FramePeriod", "GigE Camera in"=w500) -> ("error out"=w509:errorcluster, "Attribute Variant"=w508:variant)  [unwired: 5 in, 2 out]
            n232 = Compound Arithmetic op=MULTIPLY(w526, w525, w524) -> (w523:dbl)
            n233 = call "Variant to Data.vim"("variant"=w516, "type"=0.0, "Error In"=w517) -> ("data"=→"FrameRate":dbl, "Error Out"=w515:errorcluster)  [unwired: 11 in]
            n234 = call "Variant to Data.vim"("variant"=w508, "type"=i64 0, "Error In"=w509) -> ("data"=w505:i64, "Error Out"=w506:errorcluster)  [unwired: 11 in]
            n235 = local write "Traversal [mm]"(w523) -> ()
            n236 = property on="FramePeriod" class="DigNum (strict)"(error in=w506, "Value"=w505) -> (error out=w504:errorcluster)  [unwired: 1 in, 1 out]
            n237 = Merge Errors(w515, w504) -> (w503:errorcluster)
          }
          frame Default {
            # "UNKNOWN COMMAND"
            n238 = Concatenate Strings("Unkown Command: ", w534) -> (w533:string)
            n239 = call <vilib>:"Error Cluster From Error Code.vi"("error in (no error)"=w537, "error message (\"\")"=w533, "error code (0)"=5001) -> ("error out"=w536:errorcluster)  [unwired: 6 in]
          }
        }
      }
      frame True {
        # "Worker Cases Burst"
        n240 = case shown="\"Grab\"" w548 {
          selector: w548 -> [w568 w575]
          tunnel: w550 -> [w565 w574]
          tunnel: [w559 w574] -> w549
          tunnel: [w568 w575] -> w547
          tunnel: w546 -> [w564 w573]
          tunnel: [w553 w573] -> w545
          tunnel: [0 ("repeat") -1 ("repeat")] -> w544
          tunnel: [_ w571] -> w543
          frame "Grab" {
            n241 = call-dynamic "Do Grab Acquisition.vi"("error in (no error)"=w565, "GigE Camera in"=w564) -> ("error out"=w563:errorcluster, "Acquired Frames per Second"=→"Acquired FPS":dbl, "GigE Camera out"=w554:refnum<class "C5.lvclass">, "Processed Frames per Second"=→"Processed FPS":dbl)  [unwired: 5 in, 1 out]
            n242 = local read "2D Mode Camsettings"() -> (w552:T4)
            n243 = call "Get Vertical Flipped Image.vi"("error in (no error)"=w563, "C5 in"=w554) -> ("error out"=w560:errorcluster, "Vertically Flipped Pixels (U16)"=w566:u16[][], "C5 out"=w553:refnum<class "C5.lvclass">)  [unwired: 7 in]
            n244 = Transpose 2D Array(2D array=w566) -> (transposed array=w558:u16[][])
            "Intensity Image" <- w558
            n245 = control-ref of="2D Detail Graph"() -> (w556:refnum<vi>)
            n246 = control-ref of="Intensity Image"() -> (w557:refnum<vi>)
            n247 = Unbundle By Name(w552) -> ("AOIThreshold"=w551:dbl)
            n248 = call "Graph under Cursor (SubVI).vi"("AOIThreshold"=w551, "error in (no error)"=w560, "Detail Graph"=w556, "Intensity Graph"=w557, "Intensity Image"=w558) -> ("error out"=w559:errorcluster, "Intensity under Cursor"=w555:u16[][])  [unwired: 5 in]
            n249 = local write "2D Detail Graph"(w555) -> ()
          }
          frame Default {
            n250 = call-poly "Enqueue Message Poly.vi"("Message Data"="Warning: Unknown Burst State" ("Message"), "Message"="Log") -> ("channel"=w571:T1)  [unwired: 9 in]
          }
        }
      }
    }
    n251 = call "Error Handler - Message Handling Loop.vi"("channel"=w91, "error in (no error)"=w81, "Shutdown?"=w90) -> ("dup error in"=w88:errorcluster, "Shutdown!"=w89:bool)  [unwired: 7 in]
  }
  "error out" <- w11
  "remote response" <- w1
